vi "error-check.vi"(1 "error-array":errorcluster[](array[cluster])) -> (0 "error-strings":string[](array[string]))   [LabVIEW 2017, in "NI_fuzzy logic.lvlib"]
uses:
  <vilib>/addons/control/fuzzy/NI_fuzzy logic.lvlib
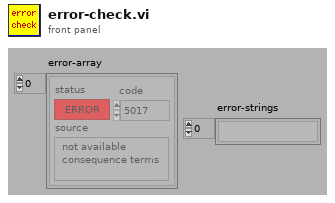
[diagram p1: front panel]
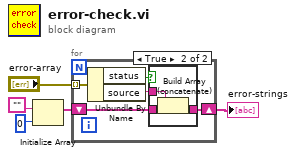
[diagram p0: block diagram]
diagram:
  n1 = Initialize Array("", 0) -> (w3:string[])
  n2 = for {
    tunnel: "error-array" -> [w10] mode=indexing
    shift-right: [w7] -> w1
    shift-left: w3 -> [w8]
    n3 = Unbundle By Name(w10) -> ("status"=w9:bool, "source"=w6:string)
    n4 = case shown="True" w9 {
      tunnel: w8 -> [w11 w14]
      tunnel: [w11 w13] -> w7
      tunnel: w6 -> [_ w12]
      frame False {
      }
      frame True {
        n5 = Build Array (concatenate)(w12, w14) -> (w13:string[])
      }
    }
  }
  "error-strings" <- w1
